vi "LSM9DS1_RefNum Registry Set.vi"(8 "error in (no error)":errorcluster, 10 "refnum name":string="My Gyro RefNum", 11 "LSM9DS1DevRef":T1={"DevStatus"={"status"=FALSE, "code"=0, "source"=""}, "Gyro Offset"={"Xzero"=0.0, "Yzero"=0.0, "Zzero"=0.0}, "StdDev Rates"={"Xsdo"=0.0, "Ysdo"=0.0, "Zsdo"=0.0}, "Reset"=FALSE, "Accel Offset"={"Xzero"=0.0, "Yzero"=0.0, "Zzero"=0.0}, "Motion Thresh"=0.0, "Mag Offset"={"Xzero"=1.0, "Yzero"=1.0, "Zzero"=1.0}, "I2C Bus"=enum."I2C On-Board", "Handle"=0, "Anomaly Thresh"=0.0, "Local Mag"=0.0, "Accel/Gyro_Address"=enum."0x6A", "Accel_Range"=enum."±2g", "Gyro_Range"=enum."±245dps", "Mag_Range"=enum."±2 gauss", "Mag_Address"=enum."0x1C", "accel_active"=FALSE, "gyro_active"=FALSE, "mag_active"=FALSE}) -> (0 "error out":errorcluster, 3 "LSM9DS1DevRef Out":T1={"DevStatus"={"status"=FALSE, "code"=0, "source"=""}, "Gyro Offset"={"Xzero"=0.0, "Yzero"=0.0, "Zzero"=0.0}, "StdDev Rates"={"Xsdo"=0.0, "Ysdo"=0.0, "Zsdo"=0.0}, "Reset"=FALSE, "Accel Offset"={"Xzero"=0.0, "Yzero"=0.0, "Zzero"=0.0}, "Motion Thresh"=0.0, "Mag Offset"={"Xzero"=1.0, "Yzero"=1.0, "Zzero"=1.0}, "I2C Bus"=enum."I2C On-Board", "Handle"=0, "Anomaly Thresh"=0.0, "Local Mag"=0.0, "Accel/Gyro_Address"=enum."0x6A", "Accel_Range"=enum."±2g", "Gyro_Range"=enum."±245dps", "Mag_Range"=enum."±2 gauss", "Mag_Address"=enum."0x1C", "accel_active"=FALSE, "gyro_active"=FALSE, "mag_active"=FALSE})   [LabVIEW 2015]
doc: "Sets a reference into a registry so that other VIs can call the reference. After you set a reference, you can call that reference with the RefNum Registry Get VI."
uses:
  LSM9DS1DevRef.ctl
  <vilib>/Rock Robotics/SystemInterfaces/i2clib/i2c_bus.ctl
  <vilib>/Rock Robotics/WPI/Utilities/Refnum Registry Operation.ctl
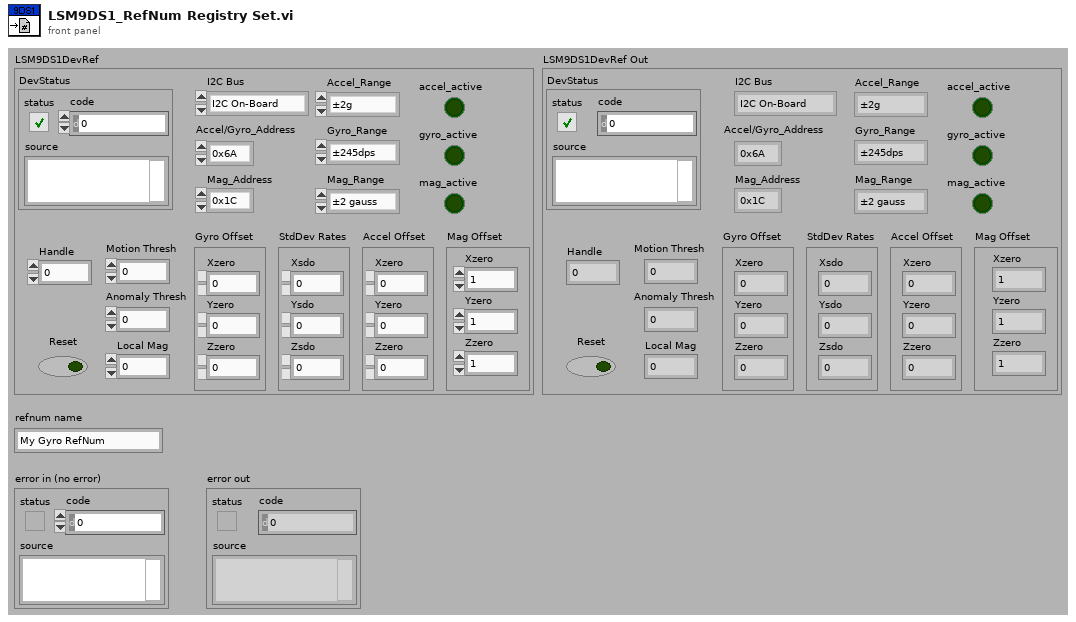
[diagram p1: front panel]
types:
  T1 = typedef "LSM9DS1DevRef.ctl" = cluster{"DevStatus":errorcluster, "Gyro Offset":cluster{"Xzero":dbl, "Yzero":dbl, "Zzero":dbl}, "StdDev Rates":cluster{"Xsdo":dbl, "Ysdo":dbl, "Zsdo":dbl}, "Reset":bool, "Accel Offset":cluster{"Xzero":dbl, "Yzero":dbl, "Zzero":dbl}, "Motion Thresh":dbl, "Mag Offset":cluster{"Xzero":dbl, "Yzero":dbl, "Zzero":dbl}, "I2C Bus":T2, "Handle":i32, "Anomaly Thresh":dbl, "Local Mag":dbl, "Accel/Gyro_Address":enum8{"0x6A", "0x6B"}, "Accel_Range":enum16{"±2g", "±16g", "±4g", "±8g", "disabled"}, "Gyro_Range":enum16{"±245dps", "±500dps", "disabled", "±2000dps"}, "Mag_Range":enum16{"±2 gauss", "±4 gauss", "±8 gauss", "±16 gauss", "disabled"}, "Mag_Address":enum8{"0x1C", "0x1E"}, "accel_active":bool, "gyro_active":bool, "mag_active":bool}
  T2 = typedef "i2c_bus.ctl" = enum16{"I2C On-Board", "I2C MXP", "Invalid"}
  T3 = typedef "Refnum Registry Operation.ctl" = enum16{"set", "get", "delete", "get all names", "read name"}
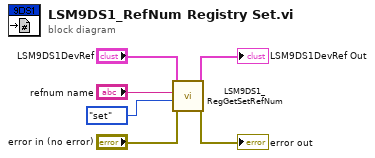
[diagram p0: block diagram]
diagram:
  n1 = call "LSM9DS1_RegGetSetRefNum.vi"("error in (no error)"="error in (no error)", "Operation"=Refnum_Registry_Operation."set" ("menu"), "refnum name"="refnum name", "LSM9DS1DevRef"="LSM9DS1DevRef") -> ("error out"=→"error out":errorcluster, "LSM9DS1DevRef Out"=→"LSM9DS1DevRef Out":T1)  [unwired: 6 in]
